vi "3.8-TCP Data Server.vi"() -> ()   [LabVIEW 2010]
doc: "Sends a specified waveform through a TCP port. The VI first listens for a connection and, once established, sends the number of bytes to be sent followed by the data. After the data is sent, the VI waits for an 'all received' signal from the client and then breaks the connection.\n\n<B>Note:</B> Requires the Data Client.vi located in the same library as this VI."
uses:
  3.0 Flow Control/3.0 List of Loops.ctl
  3.0-Global.vi
panel:
  in  "Port":u16=33483 min=1025 step=1
  # "Instructions:\n1. Open the Data Client.vi\n2. Run This VI first.\n3. Run the Data Client.vi Second.\n4. Adjust the # of Points Function, and Noise Level controls.\n5. Observe the Chart on the Data Client.vi.\n6. Stop This VI. The Data Client.vi will time out and stop."
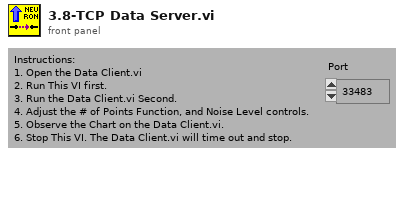
[diagram p1: front panel]
types:
  T1 = typedef "3.0 List of Loops.ctl" = enum16{"3.0 State Update", "3.0 GUI", "3.1 Act", "3.1 4.7.1 Act UDP", "3.1 Joystick", "3.2 Where", "3.2.0 Kalman Filter", "3.2 4.7.2 Where UDP", "3.3 What", "3.3 4.7.3 What UDP", "3.4 How", "3.4 4.7.4 How UDP", "3.5 Limbic", "3.8 TCP", "3.6 Cerebellum", "3.8 TCP Act"}
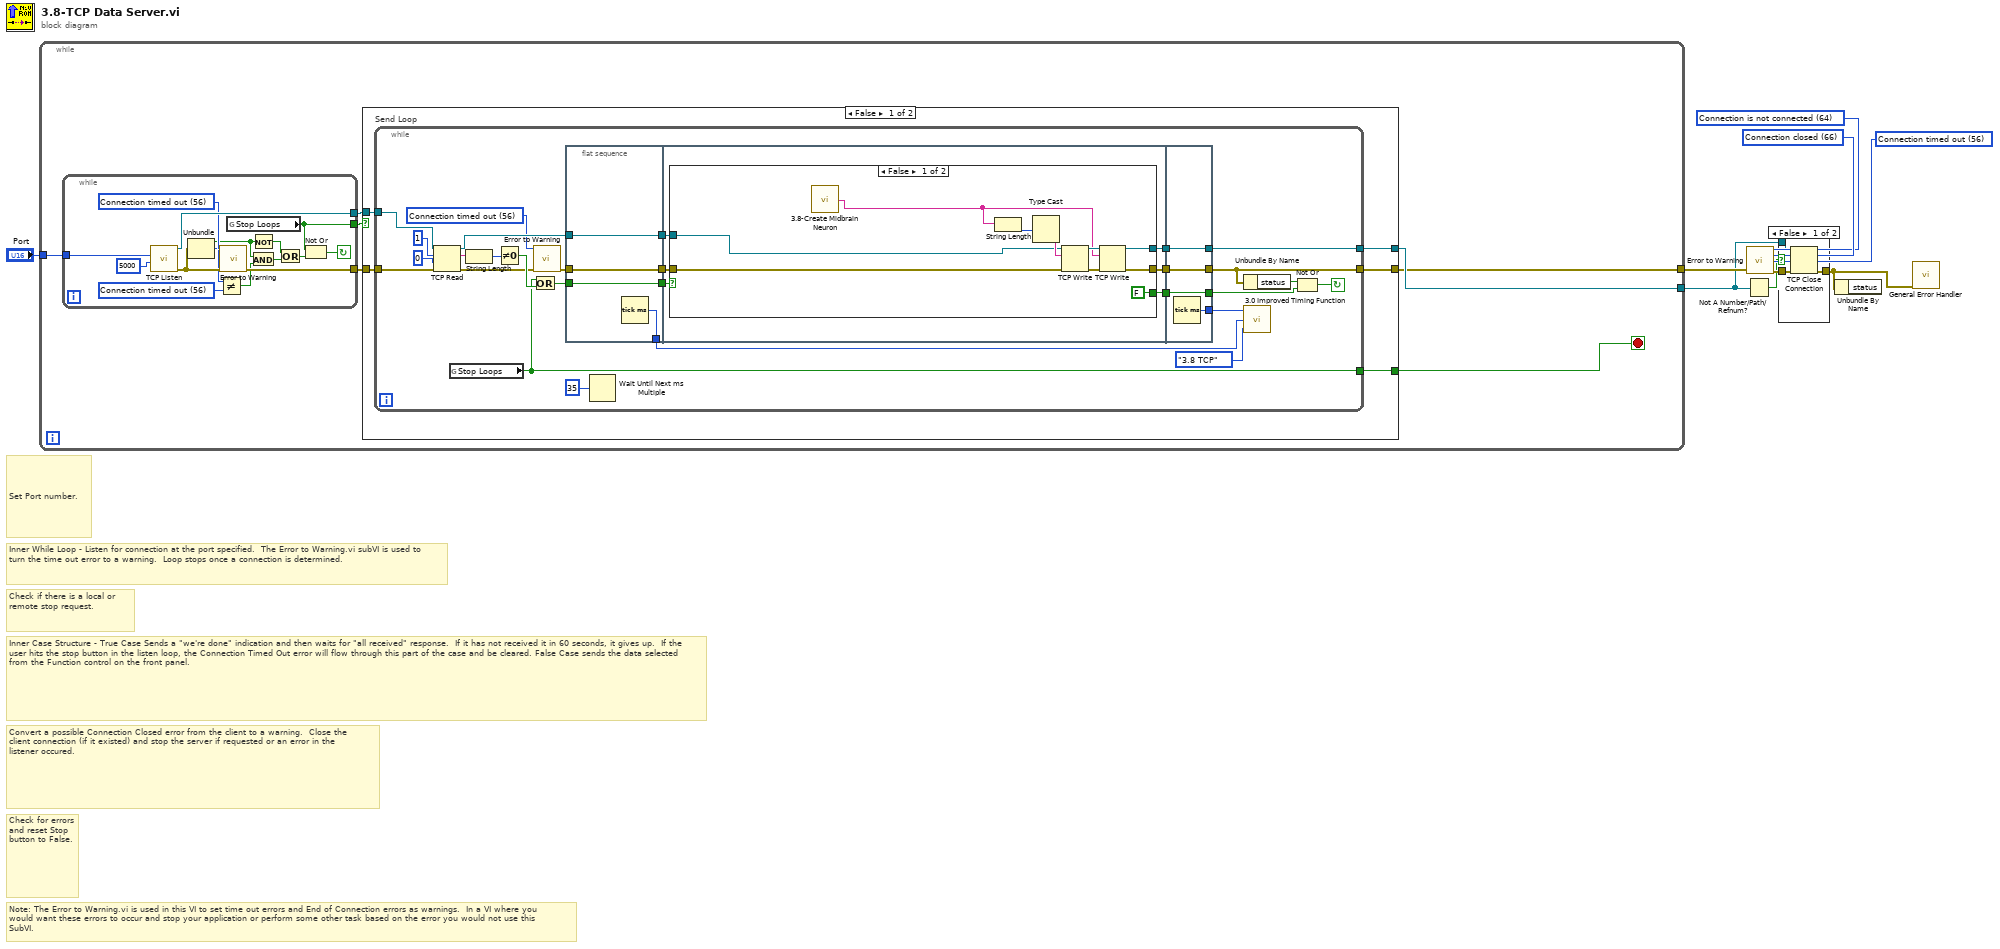
[diagram p0: block diagram]
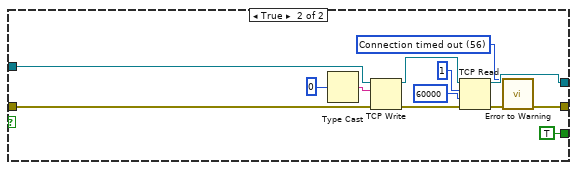
[diagram p3: hidden frame]
diagram:
  w8 = 56 items=["No Error", "Argument Error", "Memory Full", "Out of Zone", "End of File", "File Already Open", "Generic File IO Error", "File Not Found", "File Permission Error", "Disk Full", "Duplicate Path", "Too Many Files Open", "Not Enabled", "Resource File Not Found", "Cannot Add Resource", "Resource Not Found", "Image Not Found", "Image Memory Error", "Pen Does Not Exist", "Config Bad Type", "Config Token Not Found", "Config Parse Error", "Config Memory Error", "Bad External Code Format", "Bad External Code Offset", "External Code Not Present", "Null Window", "Destroy Window Mixup", "Null Menu", "Print Aborted", "Bad Print Record", "Print Driver Error", "Windows Error During Print", "Memory Error During Print", "Print Dialog Error", "Generic Print Error", "Invalid Device Refnum", "Device Not Found", "Device Parameter Error", "Device Unit Error", "Can't Open Device", "Device Call Aborted", "Generic Error", "Cancelled By User", "Object ID Too Low", "Object ID Too High", "Object Not In Heap", "Unknown Heap", "Bad DefProc ID", "DefProc Not In Table", "Message Out Of Range", "Null Method", "Unknown Message", "Manager Call Not Supported", "Bad address", "Connection In progress", "Connection timed out", "Connection is already in progress", "Network attribute not supported", "Network error", "Address in use", "System out of memory", "Connection aborted", "Connection refused", "Connection is not connected", "Connection is already connected", "Connection closed", "Initialize error (interapplication manager)", "Bad occurrence", "Wait on unbound occurrence handler", "Occurrence queue overflow", "Bad path", "Semaphore not signaled", "Unrecognized type (interapplication manager)"] ("3rd Error to Convert")
  w6 = 66 items=["No Error", "Argument Error", "Memory Full", "Out of Zone", "End of File", "File Already Open", "Generic File IO Error", "File Not Found", "File Permission Error", "Disk Full", "Duplicate Path", "Too Many Files Open", "Not Enabled", "Resource File Not Found", "Cannot Add Resource", "Resource Not Found", "Image Not Found", "Image Memory Error", "Pen Does Not Exist", "Config Bad Type", "Config Token Not Found", "Config Parse Error", "Config Memory Error", "Bad External Code Format", "Bad External Code Offset", "External Code Not Present", "Null Window", "Destroy Window Mixup", "Null Menu", "Print Aborted", "Bad Print Record", "Print Driver Error", "Windows Error During Print", "Memory Error During Print", "Print Dialog Error", "Generic Print Error", "Invalid Device Refnum", "Device Not Found", "Device Parameter Error", "Device Unit Error", "Can't Open Device", "Device Call Aborted", "Generic Error", "Cancelled By User", "Object ID Too Low", "Object ID Too High", "Object Not In Heap", "Unknown Heap", "Bad DefProc ID", "DefProc Not In Table", "Message Out Of Range", "Null Method", "Unknown Message", "Manager Call Not Supported", "Bad address", "Connection In progress", "Connection timed out", "Connection is already in progress", "Network attribute not supported", "Network error", "Address in use", "System out of memory", "Connection aborted", "Connection refused", "Connection is not connected", "Connection is already connected", "Connection closed", "Initialize error (interapplication manager)", "Bad occurrence", "Wait on unbound occurrence handler", "Occurrence queue overflow", "Bad path", "Semaphore not signaled", "Unrecognized type (interapplication manager)"] ("2nd Error to Convert")
  w5 = 64 items=["No Error", "Argument Error", "Memory Full", "Out of Zone", "End of File", "File Already Open", "Generic File IO Error", "File Not Found", "File Permission Error", "Disk Full", "Duplicate Path", "Too Many Files Open", "Not Enabled", "Resource File Not Found", "Cannot Add Resource", "Resource Not Found", "Image Not Found", "Image Memory Error", "Pen Does Not Exist", "Config Bad Type", "Config Token Not Found", "Config Parse Error", "Config Memory Error", "Bad External Code Format", "Bad External Code Offset", "External Code Not Present", "Null Window", "Destroy Window Mixup", "Null Menu", "Print Aborted", "Bad Print Record", "Print Driver Error", "Windows Error During Print", "Memory Error During Print", "Print Dialog Error", "Generic Print Error", "Invalid Device Refnum", "Device Not Found", "Device Parameter Error", "Device Unit Error", "Can't Open Device", "Device Call Aborted", "Generic Error", "Cancelled By User", "Object ID Too Low", "Object ID Too High", "Object Not In Heap", "Unknown Heap", "Bad DefProc ID", "DefProc Not In Table", "Message Out Of Range", "Null Method", "Unknown Message", "Manager Call Not Supported", "Bad address", "Connection In progress", "Connection timed out", "Connection is already in progress", "Network attribute not supported", "Network error", "Address in use", "System out of memory", "Connection aborted", "Connection refused", "Connection is not connected", "Connection is already connected", "Connection closed", "Initialize error (interapplication manager)", "Bad occurrence", "Wait on unbound occurrence handler", "Occurrence queue overflow", "Bad path", "Semaphore not signaled", "Unrecognized type (interapplication manager)"] ("1st Error to Convert")
  # "Check for errors\nand reset Stop \nbutton to False."
  # "Inner Case Structure - True Case Sends a \"we're done\" indication and then waits for \"all received\" response.  If it has not received it in 60 seconds, it gives up.  If the user hits the stop button in the listen loop, the Connection Timed Out error will flow through this part of the case and be cleared. False Case sends the data selected from the Function control on the front panel."
  # "Check if there is a local or remote stop request."
  # "Set Port number."
  # "Inner While Loop - Listen for connection at the port specified.  The Error to Warning.vi subVI is used to turn the time out error to a warning.  Loop stops once a connection is determined."
  # "Note: The Error to Warning.vi is used in this VI to set time out errors and End of Connection errors as warnings.  In a VI where you would want these errors to occur and stop your application or perform some other task based on the error you would not use this SubVI."
  # "Convert a possible Connection Closed error from the client to a warning.  Close the client connection (if it existed) and stop the server if requested or an error in the listener occured."
  n1 = while {
    tunnel: "Port" -> [w16]
    tunnel: [w11] -> w1
    tunnel: [w10] -> w2
    stop <- w12 stop-if-true
    n2 = while {
      tunnel: [w17] -> w13
      tunnel: [w26] -> w14
      tunnel: [w30] -> w15
      tunnel: w16 -> [w31]
      stop <- w28 continue-if-true
      w24 = 56 items=["No Error", "Argument Error", "Memory Full", "Out of Zone", "End of File", "File Already Open", "Generic File IO Error", "File Not Found", "File Permission Error", "Disk Full", "Duplicate Path", "Too Many Files Open", "Not Enabled", "Resource File Not Found", "Cannot Add Resource", "Resource Not Found", "Image Not Found", "Image Memory Error", "Pen Does Not Exist", "Config Bad Type", "Config Token Not Found", "Config Parse Error", "Config Memory Error", "Bad External Code Format", "Bad External Code Offset", "External Code Not Present", "Null Window", "Destroy Window Mixup", "Null Menu", "Print Aborted", "Bad Print Record", "Print Driver Error", "Windows Error During Print", "Memory Error During Print", "Print Dialog Error", "Generic Print Error", "Invalid Device Refnum", "Device Not Found", "Device Parameter Error", "Device Unit Error", "Can't Open Device", "Device Call Aborted", "Generic Error", "Cancelled By User", "Object ID Too Low", "Object ID Too High", "Object Not In Heap", "Unknown Heap", "Bad DefProc ID", "DefProc Not In Table", "Message Out Of Range", "Null Method", "Unknown Message", "Manager Call Not Supported", "Bad address", "Connection In progress", "Connection timed out", "Connection is already in progress", "Network attribute not supported", "Network error", "Address in use", "System out of memory", "Connection aborted", "Connection refused", "Connection is not connected", "Connection is already connected", "Connection closed", "Initialize error (interapplication manager)", "Bad occurrence", "Wait on unbound occurrence handler", "Occurrence queue overflow", "Bad path", "Semaphore not signaled", "Unrecognized type (interapplication manager)"] ("1st Error to Convert")
      w25 = 56 items=["No Error", "Argument Error", "Memory Full", "Out of Zone", "End of File", "File Already Open", "Generic File IO Error", "File Not Found", "File Permission Error", "Disk Full", "Duplicate Path", "Too Many Files Open", "Not Enabled", "Resource File Not Found", "Cannot Add Resource", "Resource Not Found", "Image Not Found", "Image Memory Error", "Pen Does Not Exist", "Config Bad Type", "Config Token Not Found", "Config Parse Error", "Config Memory Error", "Bad External Code Format", "Bad External Code Offset", "External Code Not Present", "Null Window", "Destroy Window Mixup", "Null Menu", "Print Aborted", "Bad Print Record", "Print Driver Error", "Windows Error During Print", "Memory Error During Print", "Print Dialog Error", "Generic Print Error", "Invalid Device Refnum", "Device Not Found", "Device Parameter Error", "Device Unit Error", "Can't Open Device", "Device Call Aborted", "Generic Error", "Cancelled By User", "Object ID Too Low", "Object ID Too High", "Object Not In Heap", "Unknown Heap", "Bad DefProc ID", "DefProc Not In Table", "Message Out Of Range", "Null Method", "Unknown Message", "Manager Call Not Supported", "Bad address", "Connection In progress", "Connection timed out", "Connection is already in progress", "Network attribute not supported", "Network error", "Address in use", "System out of memory", "Connection aborted", "Connection refused", "Connection is not connected", "Connection is already connected", "Connection closed", "Initialize error (interapplication manager)", "Bad occurrence", "Wait on unbound occurrence handler", "Occurrence queue overflow", "Bad path", "Semaphore not signaled", "Unrecognized type (interapplication manager)"] ("1st Error to Convert")
      n3 = call <vilib>:"TCP Listen.vi"("timeout ms (wait forever: -1)"=5000, "port"=w31) -> ("error out"=w27:errorcluster, "connection ID"=w30:refnum<k5>)  [unwired: 6 in, 2 out]
      n4 = Unbundle(w27) -> ("status"=w22:bool, "code"=w23:i32)  [unwired: 1 out]
      n5 = Not Equal?(x=w23, y=w24) -> (x != y?=w21:bool)
      n6 = call <vilib>:"Error to Warning.vi"("1st Error to Convert"=w25, "error in"=w27) -> ("warning out"=w26:errorcluster)  [unwired: 13 in]
      n7 = global read "3.0-Global.vi" "Stop Loops"() -> (w17:bool)
      n8 = Not(x=w22) -> (.not. x?=w20:bool)
      n9 = And(x=w22, y=w21) -> (x .and. y?=w19:bool)
      n10 = Or(x=w20, y=w19) -> (x .or. y?=w18:bool)
      n11 = Not Or(1:w18, 2:w17) -> (0:w28:bool)
    }
    n12 = case shown="False" w13 {
      selector: w13 -> [_ w102]
      tunnel: [w32 w103] -> w10
      tunnel: w15 -> [w34 w104]
      tunnel: w14 -> [w33 w103]
      tunnel: [w36 w104] -> w11
      tunnel: [w35 w102] -> w12
      frame False {
        n13 = while "Send Loop" {
          tunnel: [w47] -> w35
          tunnel: w33 -> [w61]
          tunnel: [w52] -> w32
          tunnel: [w57] -> w36
          tunnel: w34 -> [w60]
          stop <- w64 continue-if-true
          w50 = 56 items=["No Error", "Argument Error", "Memory Full", "Out of Zone", "End of File", "File Already Open", "Generic File IO Error", "File Not Found", "File Permission Error", "Disk Full", "Duplicate Path", "Too Many Files Open", "Not Enabled", "Resource File Not Found", "Cannot Add Resource", "Resource Not Found", "Image Not Found", "Image Memory Error", "Pen Does Not Exist", "Config Bad Type", "Config Token Not Found", "Config Parse Error", "Config Memory Error", "Bad External Code Format", "Bad External Code Offset", "External Code Not Present", "Null Window", "Destroy Window Mixup", "Null Menu", "Print Aborted", "Bad Print Record", "Print Driver Error", "Windows Error During Print", "Memory Error During Print", "Print Dialog Error", "Generic Print Error", "Invalid Device Refnum", "Device Not Found", "Device Parameter Error", "Device Unit Error", "Can't Open Device", "Device Call Aborted", "Generic Error", "Cancelled By User", "Object ID Too Low", "Object ID Too High", "Object Not In Heap", "Unknown Heap", "Bad DefProc ID", "DefProc Not In Table", "Message Out Of Range", "Null Method", "Unknown Message", "Manager Call Not Supported", "Bad address", "Connection In progress", "Connection timed out", "Connection is already in progress", "Network attribute not supported", "Network error", "Address in use", "System out of memory", "Connection aborted", "Connection refused", "Connection is not connected", "Connection is already connected", "Connection closed", "Initialize error (interapplication manager)", "Bad occurrence", "Wait on unbound occurrence handler", "Occurrence queue overflow", "Bad path", "Semaphore not signaled", "Unrecognized type (interapplication manager)"] ("1st Error to Convert")
          n14 = TCP Read(connection ID=w60, bytes to read=1, error in (no error)=w61, 9:0) -> (connection ID out=w58:refnum<k5>, data out=w59:string, error out=w49:errorcluster)  [unwired: 1 in]
          n15 = global read "3.0-Global.vi" "Stop Loops"() -> (w47:bool)
          n16 = String Length(string=w59) -> (length=w55:i32)
          n17 = Not Equal To 0?(x=w55) -> (x != 0?=w54:bool)
          n18 = Or(x=w47, y=w54) -> (x .or. y?=w53:bool)
          n19 = call <vilib>:"Error to Warning.vi"("1st Error to Convert"=w50, "error in"=w49) -> ("warning out"=w48:errorcluster)  [unwired: 13 in]
          n20 = flat-sequence {
            tunnel: w48 -> [w66]
            tunnel: w53 -> [w67]
            tunnel: w58 -> [w68]
            tunnel: [w68] -> w43
            tunnel: [w67] -> w42
            tunnel: [w66] -> w41
            tunnel: [w65] -> w38
            tunnel: [w73] -> w46
            tunnel: [w72] -> w45
            tunnel: [w70] -> w44
            tunnel: w43 -> [w74]
            tunnel: w42 -> [w71]
            tunnel: w41 -> [w69]
            tunnel: [w99] -> w52
            tunnel: [w100] -> w56
            tunnel: [w101] -> w57
            tunnel: w46 -> [w101]
            tunnel: w45 -> [w100]
            tunnel: w44 -> [w99]
            tunnel: [w98] -> w39
            frame #0 {
              n21 = Tick Count (ms)() -> (millisecond timer value=w65:u32)
            }
            frame #1 {
              n22 = case shown="False" w71 {
                tunnel: w69 -> [w77 w93]
                tunnel: w74 -> [w76 w91]
                tunnel: [w79 w95] -> w73
                tunnel: [w78 w86] -> w70
                tunnel: [FALSE TRUE] -> w72
                frame False {
                  n23 = call "3.8-Create Midbrain Neuron.vi"() -> ("data string"=w75:string)
                  n24 = String Length(string=w75) -> (length=w83:i32)
                  n25 = Type Cast(x=w83) -> (*(type *) &x=w82:string)  [unwired: 1 in]
                  n26 = TCP Write(connection ID=w76, data in=w82, error in (no error)=w77) -> (connection ID out=w80:refnum<k5>, error out=w81:errorcluster)  [unwired: 1 in, 1 out]
                  n27 = TCP Write(connection ID=w80, data in=w75, error in (no error)=w81) -> (connection ID out=w79:refnum<k5>, error out=w78:errorcluster)  [unwired: 1 in, 1 out]
                }
                frame True {
                  w85 = 56 items=["No Error", "Argument Error", "Memory Full", "Out of Zone", "End of File", "File Already Open", "Generic File IO Error", "File Not Found", "File Permission Error", "Disk Full", "Duplicate Path", "Too Many Files Open", "Not Enabled", "Resource File Not Found", "Cannot Add Resource", "Resource Not Found", "Image Not Found", "Image Memory Error", "Pen Does Not Exist", "Config Bad Type", "Config Token Not Found", "Config Parse Error", "Config Memory Error", "Bad External Code Format", "Bad External Code Offset", "External Code Not Present", "Null Window", "Destroy Window Mixup", "Null Menu", "Print Aborted", "Bad Print Record", "Print Driver Error", "Windows Error During Print", "Memory Error During Print", "Print Dialog Error", "Generic Print Error", "Invalid Device Refnum", "Device Not Found", "Device Parameter Error", "Device Unit Error", "Can't Open Device", "Device Call Aborted", "Generic Error", "Cancelled By User", "Object ID Too Low", "Object ID Too High", "Object Not In Heap", "Unknown Heap", "Bad DefProc ID", "DefProc Not In Table", "Message Out Of Range", "Null Method", "Unknown Message", "Manager Call Not Supported", "Bad address", "Connection In progress", "Connection timed out", "Connection is already in progress", "Network attribute not supported", "Network error", "Address in use", "System out of memory", "Connection aborted", "Connection refused", "Connection is not connected", "Connection is already connected", "Connection closed", "Initialize error (interapplication manager)", "Bad occurrence", "Wait on unbound occurrence handler", "Occurrence queue overflow", "Bad path", "Semaphore not signaled", "Unrecognized type (interapplication manager)"] ("1st Error to Convert")
                  n28 = Type Cast(x=0) -> (*(type *) &x=w88:string)  [unwired: 1 in]
                  n29 = TCP Write(connection ID=w91, data in=w88, error in (no error)=w93) -> (connection ID out=w90:refnum<k5>, error out=w92:errorcluster)  [unwired: 1 in, 1 out]
                  n30 = TCP Read(connection ID=w90, bytes to read=1, error in (no error)=w92, 9:60000) -> (connection ID out=w95:refnum<k5>, error out=w87:errorcluster)  [unwired: 1 in, 1 out]
                  n31 = call <vilib>:"Error to Warning.vi"("1st Error to Convert"=w85, "error in"=w87) -> ("warning out"=w86:errorcluster)  [unwired: 13 in]
                }
              }
            }
            frame #2 {
              n32 = Tick Count (ms)() -> (millisecond timer value=w98:u32)
            }
          }
          n33 = Wait Until Next ms Multiple(millisecond multiple=u32 35 ("milliseconds to wait")) -> ()  [unwired: 1 out]
          n34 = Unbundle By Name(w52) -> ("status"=w51:bool)
          n35 = call "3.0 Improved Timing Function.vi"("Loop"=3.0_List_of_Loops."3.8 TCP", "Start"=w38, "End"=w39) -> ()  [unwired: 1 in]
          n36 = Not Or(1:w56, 2:w51) -> (0:w64:bool)
        }
      }
      frame True {
      }
    }
  }
  n37 = Not A Number/Path/Refnum?(number/path/refnum=w1) -> (NaN/Path/Refnum?=w4:bool)
  n38 = call <vilib>:"Error to Warning.vi"("1st Error to Convert"=w5, "2nd Error to Convert"=w6, "3rd Error to Convert"=w8, "error in"=w2) -> ("warning out"=w7:errorcluster)  [unwired: 11 in]
  n39 = case shown="False" w4 {
    tunnel: w7 -> [w107 w108]
    tunnel: [w106 w108] -> w3
    tunnel: w1 -> [w105 _]
    frame False {
      n40 = TCP Close Connection(connection ID=w105, error in (no error)=w107) -> (error out=w106:errorcluster)  [unwired: 1 in, 1 out]
    }
    frame True {
    }
  }
  n41 = Unbundle By Name(w3) -> ()  [unwired: 1 out]
  n42 = call <vilib>:"General Error Handler.vi"("error in (no error)"=w3) -> ()  [unwired: 10 in, 5 out]
